vi "Matlab String(SubVI).vi"(9 "name":string, 10 "band touch win":u32(colorbox)=16734669, 11 "band touch loose":u32(colorbox)=7663) -> (3 "String":string)   [LabVIEW 2025]
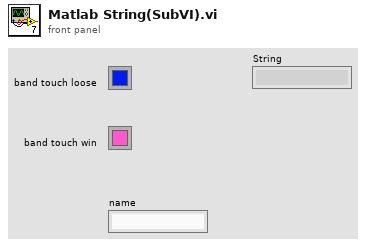
[diagram p1: front panel]
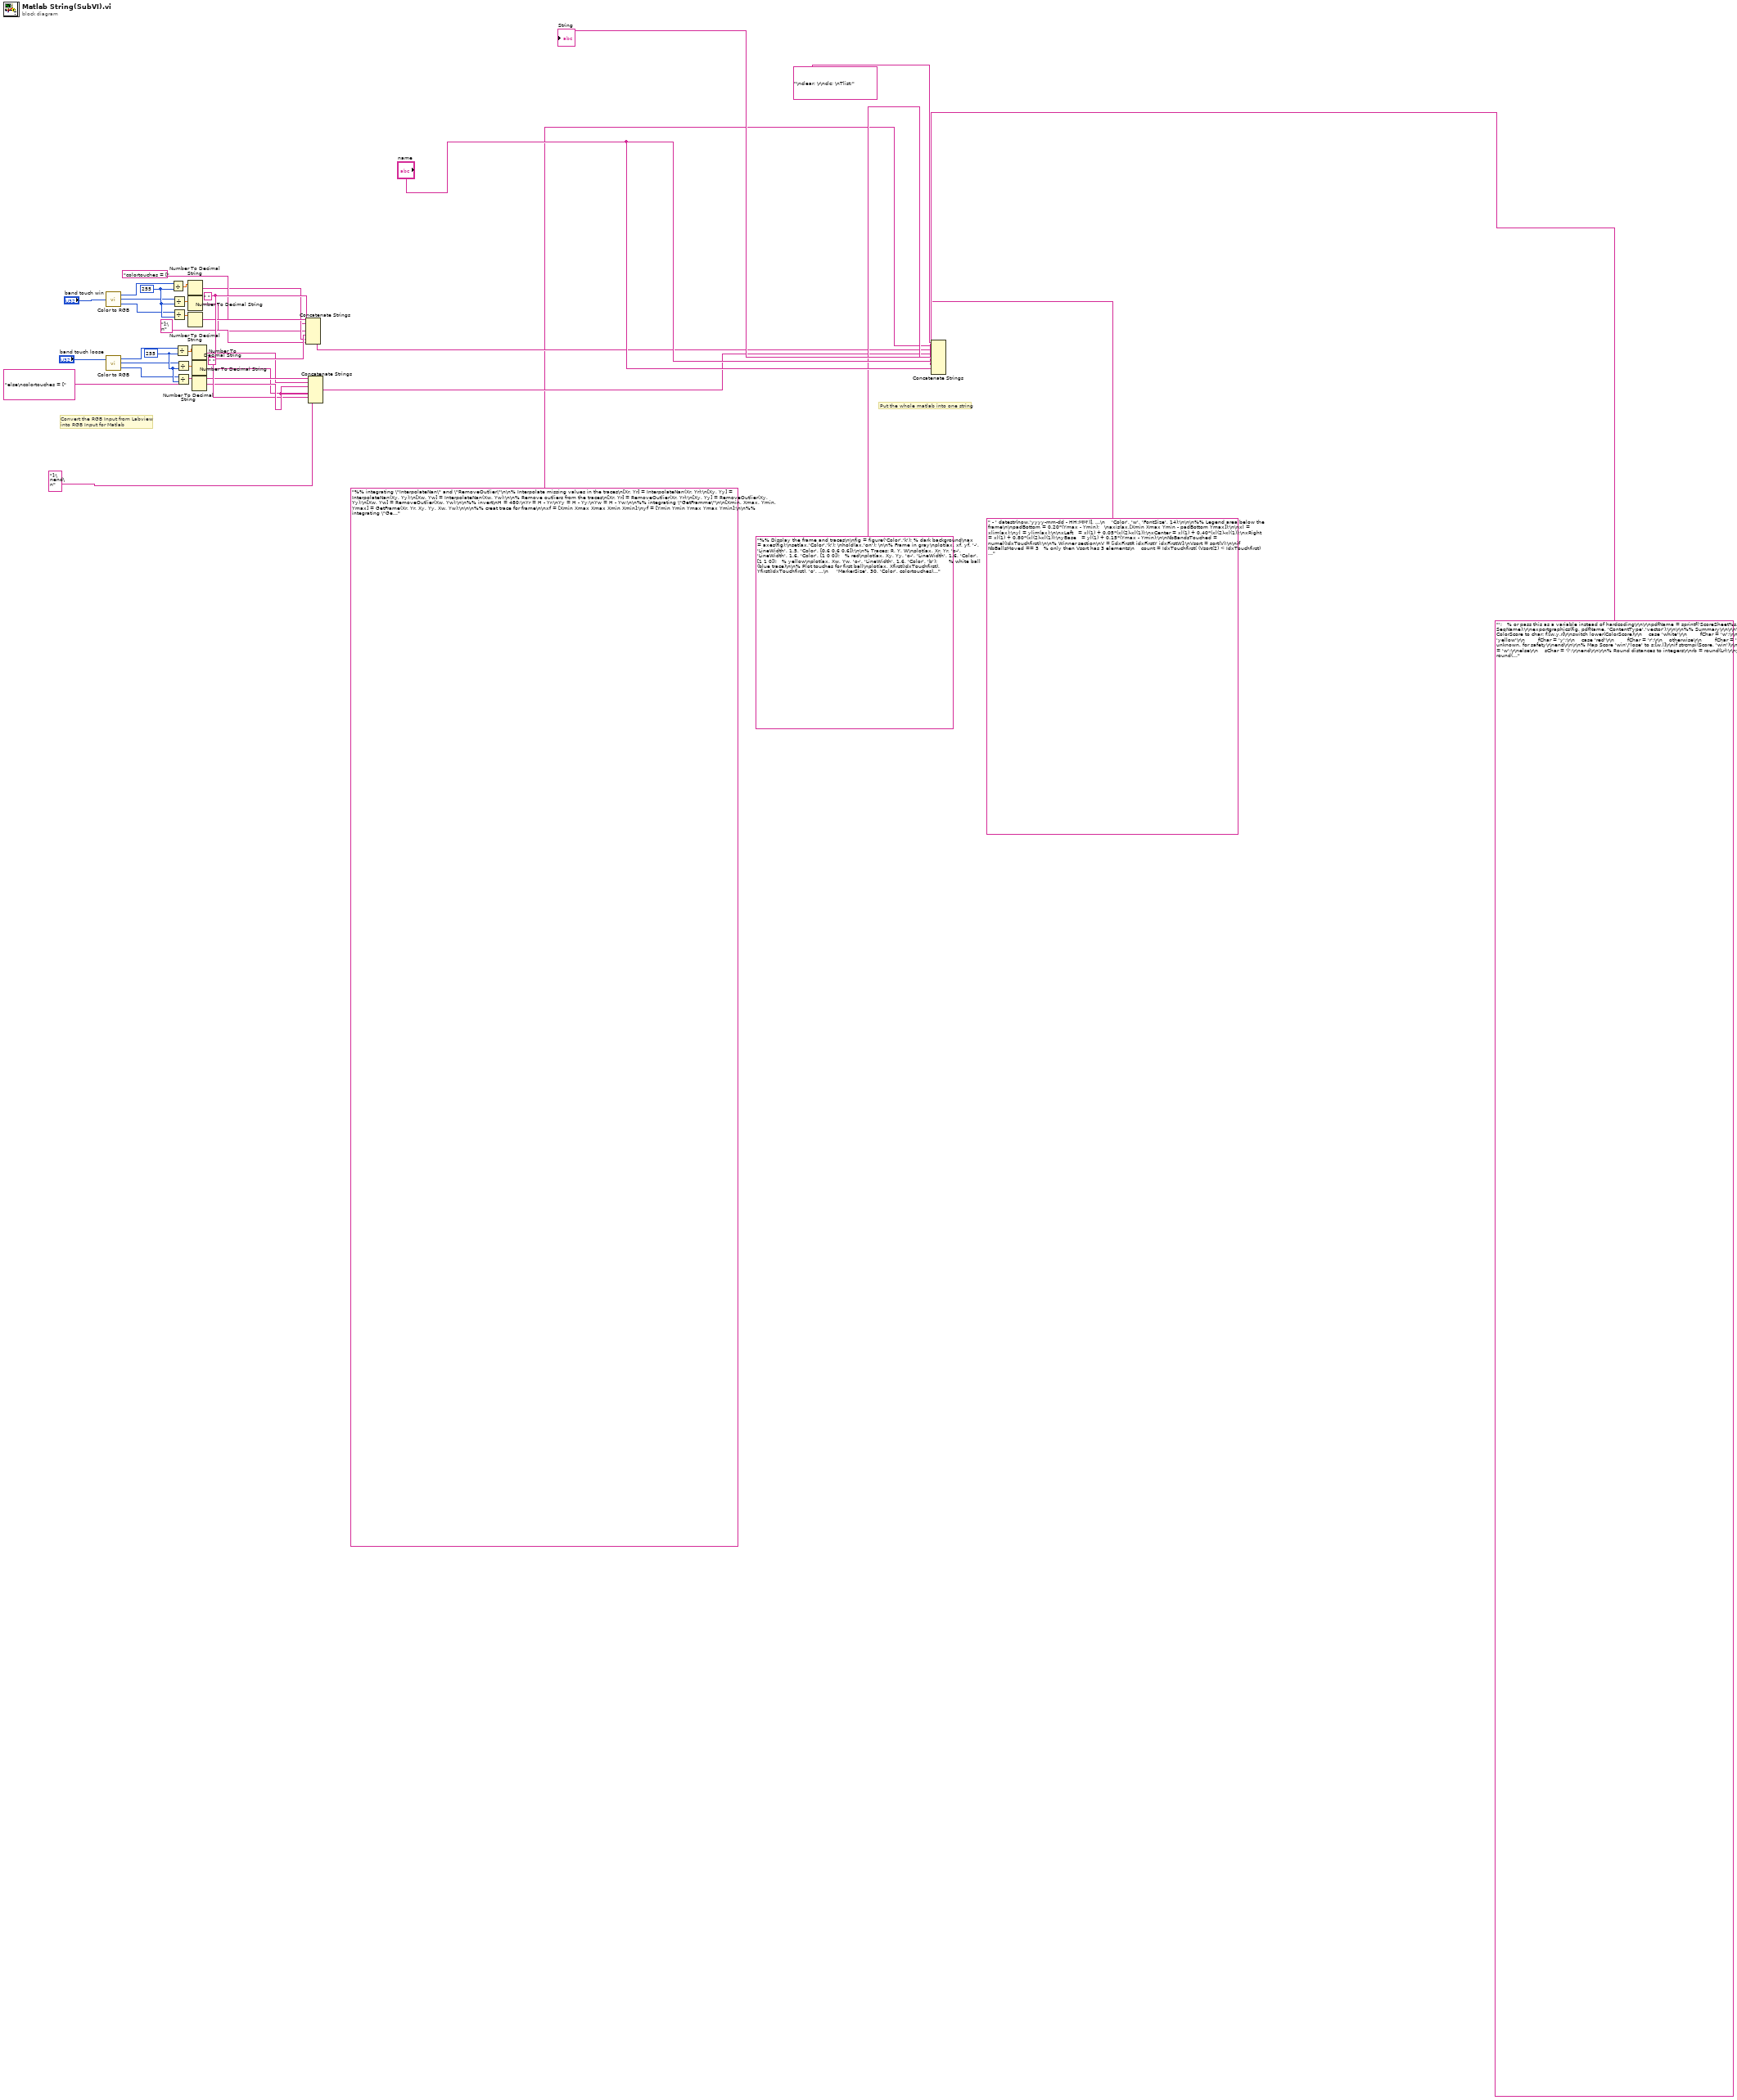
[diagram p0: block diagram]
diagram:
  w28 = " "
  w27 = 255
  w29 = " "
  w26 = 255
  # "Put the whole matlab into one string"
  # "Convert the RGB Input from Labview\ninto RGB Input for Matlab"
  n1 = call <vilib>:"Color to RGB.vi"("Color"="band touch win") -> ("R"=w22:u8, "G"=w23:u8, "B"=w24:u8)  [unwired: 1 out]
  n2 = call <vilib>:"Color to RGB.vi"("Color"="band touch loose") -> ("R"=w3:u8, "G"=w4:u8, "B"=w5:u8)  [unwired: 1 out]
  n3 = Divide(x=w22, y=w27) -> (x/y=w15:dbl)
  n4 = Divide(x=w23, y=w27) -> (x/y=w16:dbl)
  n5 = Divide(x=w24, y=w27) -> (x/y=w17:dbl)
  n6 = Divide(x=w3, y=w26) -> (x/y=w7:dbl)
  n7 = Divide(x=w4, y=w26) -> (x/y=w8:dbl)
  n8 = Divide(x=w5, y=w26) -> (x/y=w9:dbl)
  n9 = Number To Decimal String(number=w15) -> (decimal integer string=w18:string)  [unwired: 1 in]
  n10 = Number To Decimal String(number=w16) -> (decimal integer string=w19:string)  [unwired: 1 in]
  n11 = Number To Decimal String(number=w17) -> (decimal integer string=w20:string)  [unwired: 1 in]
  n12 = Number To Decimal String(number=w7) -> (decimal integer string=w10:string)  [unwired: 1 in]
  n13 = Number To Decimal String(number=w8) -> (decimal integer string=w11:string)  [unwired: 1 in]
  n14 = Number To Decimal String(number=w9) -> (decimal integer string=w12:string)  [unwired: 1 in]
  n15 = Concatenate Strings("colortouches = [" ("string"), w18, w28, w19, w28, w20, "];\n" ("string")) -> (w30:string)
  n16 = Concatenate Strings("else\ncolortouches = [" ("string"), w10, w29, w11, w29, w12, "];\nend\n" ("string")) -> (w31:string)
  n17 = Concatenate Strings("\nclear; \r\nclc; \nTlist;", "%% integrating \"InterpolateNan\" and \"RemoveOutlier\"\n\n% Interpolate missing values in the traces\n[Xr, Yr] = InterpolateNan(Xr, Yr);\n[Xy, Yy] = InterpolateNan(Xy, Yy);\n[Xw, Yw] = InterpolateNan(Xw, Yw);\n\n% Remove outliers from the traces\n[Xr, Yr] = RemoveOutlier(Xr, Yr);\n[Xy, Yy] = RemoveOutlier(Xy, Yy);\n[Xw, Yw] = RemoveOutlier(Xw, Yw);\n\n%% invert\nH = 480;\nYr = H - Yr;\nYy = H - Yy;\nYw = H - Yw;\n\n%% integrating \"GetFramme\"\n\n[Xmin, Xmax, Ymin, Ymax] = GetFrame(Xr, Yr, Xy, Yy, Xw, Yw);\n\n\n%% creat trace for frame\n\nxf = [Xmin Xmax Xmax Xmin Xmin];\nyf = [Ymin Ymin Ymax Ymax Ymin];\n\n%% integrating \"GetBallPathLength\" and \"GetFirstMoveIdx\"\nMoveDistPx = 9;\nLr = GetBallPathLength(Xr, Yr);\nLy = GetBallPathLength(Xy, Yy);\nLw = GetBallPathLength(Xw, Yw);\n\n[idxFirstR, DistMoveR] = GetFirstMoveIdx(Xr, Yr, MoveDistPx);\n[idxFirstY, DistMoveY] = GetFirstMoveIdx(Xy, Yy, MoveDistPx);\n[idxFirstW, DistMoveW] = GetFirstMoveIdx(Xw, Yw, MoveDistPx);\n\n%% integrating \"GetTouchIdx\" and \"GetBallMoveOrder\"\n\nBallBorderDist = 9;\nIdxTouchR = GetTouchIdx(Xr, Yr, Xmin, Xmax, Ymin, Ymax, BallBorderDist);\nIdxTouchY = GetTouchIdx(Xy, Yy, Xmin, Xmax, Ymin, Ymax, BallBorderDist);\nIdxTouchW = GetTouchIdx(Xw, Yw, Xmin, Xmax, Ymin, Ymax, BallBorderDist);\n\n[FirstBall, SecondBall, LastBall, NbBallsMoved] = GetBallMoveOrder(Xr, Yr, Xy, Yy, Xw, Yw, MoveDistPx);\n\nif FirstBall == 1\n    Xfirst = Xr;\n    Yfirst = Yr;\n    IdxTouchfirst = IdxTouchR;\n    ColorScore = 'red';\nelseif FirstBall == 2\n    Xfirst = Xy;\n    Yfirst = Yy;\n    IdxTouchfirst = IdxTouchY;\n    ColorScore = 'yellow';\nelse \n    Xfirst = Xw;\n    Yfirst = Yw;\n    IdxTouchfirst = IdxTouchW;\n    ColorScore = 'white';\nend\n\n%% determin Win/lose\n\nScore = GetWinnerScore(idxFirstR, idxFirstY, idxFirstW, IdxTouchfirst, NbBallsMoved);\n\nif strcmp(Score, 'win')\n    \n\n", w30, w31, "%% Display the frame and traces\n\nfig = figure('Color','k'); % dark background\nax = axes(fig);\nset(ax,'Color','k'); \nhold(ax,'on'); \n\n% Frame in gray\nplot(ax, xf, yf, '-', 'LineWidth', 1.5, 'Color', [0.6 0.6 0.6]);\n\n% Traces: R, Y, W\nplot(ax, Xr, Yr, 'o-', 'LineWidth', 1.6, 'Color', [1 0 0]);   % red\nplot(ax, Xy, Yy, 'o-', 'LineWidth', 1.6, 'Color', [1 1 0]);   % yellow\nplot(ax, Xw, Yw, 'o-', 'LineWidth', 1.6, 'Color', 'b');       % white ball (blue trace)\n\n% Plot touches for first ball\nplot(ax, Xfirst(IdxTouchfirst), Yfirst(IdxTouchfirst), 'o', ...\n     'MarkerSize', 30, 'Color', colortouches);\n\n% Plot origins\nplot(ax, Xr(1), Yr(1), 'hexagram', 'MarkerSize', 20, 'Color', [1 0 0]);\nplot(ax, Xy(1), Yy(1), 'hexagram', 'MarkerSize', 20, 'Color', [1 1 0]);\nplot(ax, Xw(1), Yw(1), 'hexagram', 'MarkerSize', 20, 'Color', 'b');\n\n% Design: frame sizing\naxis(ax,'equal');\naxis(ax,[Xmin Xmax Ymin Ymax]);\n\naxis(ax,'off');   \n\ntitle(ax, ['Scores sheet -", "name", " - ' datestr(now,'yyyy-mm-dd - HH:MM')], ...\n    'Color', 'w', 'FontSize', 14);\n\n\n%% Legend area below the frame\n\npadBottom = 0.20*(Ymax - Ymin);   \naxis(ax,[Xmin Xmax Ymin - padBottom Ymax]);\n\nxl = xlim(ax);\nyl = ylim(ax);\n\nxLeft   = xl(1) + 0.05*(xl(2)-xl(1));\nxCenter = xl(1) + 0.40*(xl(2)-xl(1));\nxRight  = xl(1) + 0.80*(xl(2)-xl(1));\nyBase   = yl(1) + 0.15*(Ymax - Ymin);\n\nNbBandsTouched = numel(IdxTouchfirst);\n\n% Winner section\nV = [idxFirstR idxFirstY idxFirstW];\nVsort = sort(V);\n\nif NbBallsMoved == 3   % only then Vsort has 3 elements\n    count = IdxTouchfirst( (Vsort(2) < IdxTouchfirst) & (IdxTouchfirst < Vsort(3)) );\n    NbBandsWin = numel(count);\nelse\n    NbBandsWin = 0;\nend\n\nif NbBallsMoved == 3 && NbBandsWin >= 3\n    Score = 'win';\nelse\n    Score = 'lose';\nend\n\n\ntext(xLeft, yBase, sprintf('Score sheet for \"%s\"', ColorScore), 'Color', 'w', 'FontSize', 12);\ntext(xLeft, yBase-30, sprintf('--- %s ---', Score), 'Color', 'w', 'FontSize', 12);\n\n% Distances\ntext(xLeft,   yBase-80, sprintf('red_d : %.0fpx',   Lr), 'Color', 'w', 'FontSize', 12);\ntext(xCenter, yBase-80, sprintf('yellow_d : %.0fpx', Ly), 'Color', 'w', 'FontSize', 12);\ntext(xRight,  yBase-80, sprintf('white_d : %.0fpx', Lw), 'Color', 'w', 'FontSize', 12);\n\n% Ball & band stats\ntext(xRight, yBase,   sprintf('%d ball(s) moved',   NbBallsMoved),   'Color', 'w', 'FontSize', 12);\ntext(xRight, yBase-30, sprintf('%d band(s) touched', NbBandsTouched), 'Color', 'w', 'FontSize', 12);\n\n%% PDF\nSeqName = '", "name", "';   % or pass this as a variable instead of hardcoding\r\n\r\npdfName = sprintf('ScoreSheet%s.pdf', SeqName);\r\nexportgraphics(fig, pdfName, 'ContentType','vector');\r\n\r\n%% Summary\r\n\r\n% Map ColorScore to char: f:[w,y,r]\r\nswitch lower(ColorScore)\r\n    case 'white'\r\n        fChar = 'w';\r\n    case 'yellow'\r\n        fChar = 'y';\r\n    case 'red'\r\n        fChar = 'r';\r\n    otherwise\r\n        fChar = 'x';   % unknown, for safety\r\nend\r\n\r\n% Map Score 'win'/'lose' to s:[w,l]\r\nif strcmpi(Score, 'win')\r\n    sChar = 'w';\r\nelse\r\n    sChar = 'l';\r\nend\r\n\r\n% Round distances to integers\r\nrb = round(Lr);\r\nyb = round(Ly);\r\nwb = round(Lw);\r\n\r\nsummaryStr = sprintf('f:%c; s:%c; n:%d; b:%d; rb:%d; yb:%d; wb:%d;', ...\r\n    fChar, sChar, NbBallsMoved, NbBandsTouched, rb, yb, wb);\r\n\r\nSummaryName = sprintf('Summary%s.txt', SeqName);\r\n\r\nfid = fopen(SummaryName, 'w');\r\nfprintf(fid, '%s\\n', summaryStr);\r\nfclose(fid);\r\n\r\n%% function InterpolateNan\r\n\r\nfunction [X, Y] = InterpolateNan(X, Y)\r\n\r\n    if isnan(X(1)),  X(1)  = 0; end\r\n    if isnan(X(end)),X(end)= 0; end\r\n\r\n    defX = ~isnan(X);\r\n    idX = 1:numel(X);\r\n    idx_defX = find(defX);\r\n    X =interp1(idx_defX,X(defX),idX,'next');\r\n\r\n    if isnan(Y(1)),  Y(1)  = 0; end\r\n    if isnan(Y(end)),Y(end)= 0; end\r\n\r\n    defY = ~isnan(Y);\r\n    idY = 1:numel(Y);\r\n    idx_defY = find(defY);\r\n    Y =interp1(idx_defY,Y(defY),idY,'next');\r\nend\r\n%% function RemoveOutlier\r\n\r\nfunction [X, Y] = RemoveOutlier(X, Y)\r\n    OX =isoutlier(X,'movmedian',10);\r\n    OY =isoutlier(Y,'movmedian',10);\r\n\r\n    O = OX & OY;\r\n    idx = find(O);\r\n    idx = idx(idx > 1);\r\n    \r\n    X(idx) = X(idx - 1);\r\n    Y(idx) = Y(idx - 1);\r\nend\r\n\r\n%% function GetFrame\r\n\r\nfunction [Xmin, Xmax, Ymin, Ymax] = GetFrame(Xr, Yr, Xy, Yy, Xw, Yw)\r\n    Xmin = min([Xr(:); Xy(:); Xw(:)], [], 'omitnan');\r\n    Xmax = max([Xr(:); Xy(:); Xw(:)], [], 'omitnan');\r\n    Ymin = min([Yr(:); Yy(:); Yw(:)], [], 'omitnan');\r\n    Ymax = max([Yr(:); Yy(:); Yw(:)], [], 'omitnan');\r\nend\r\n\r\n%% function GetBallPathLenght\r\n\r\nfunction PathLength = GetBallPathLength(X, Y)\r\n    dx = diff(X); \r\n    dy = diff(Y);\r\n    PathLength = sum( sqrt(dx.^2 + dy.^2) );\r\nend\r\n\r\n%% function GetFirstMoveIdx\r\n\r\nfunction [FirstMoveIdx, MoveDist] = GetFirstMoveIdx(X, Y, MoveDistPx)\r\n\r\n    X = X(:); \r\n    Y = Y(:);\r\n\r\n    % 1) Distances per segment \r\n    MoveDist = hypot(diff(X), diff(Y));     % length = N-1\r\n\r\n    % 2) Distance from initial position \r\n    DistFromStart = hypot(X - X(1), Y - Y(1));  % length = N\r\n\r\n    FirstMoveIdx = find(DistFromStart > MoveDistPx, 1, 'first');\r\n    if isempty(FirstMoveIdx)\r\n        FirstMoveIdx = [];  % as required: return [] if never moved\r\n    end\r\nend\r\n\r\n\r\n%% function GetTouchIdx\r\n\r\nfunction IdxTouch = GetTouchIdx(X, Y, Xmin, Xmax, Ymin, Ymax, BallBorderDist)\r\n%GETTOUCHIDX  Return time indices where the ball first touches a cushion.\r\n% A \"touch\" happens when the ball is closer than BallBorderDist to any\r\n% table border. Only the *first* index of each consecutive run is kept.\r\n\r\n    if nargin < 7 || isempty(BallBorderDist)      \nBallBorderDist = 9;            \r\n    end\r\n\r\n    % Ensure column vectors\r\n    X = X(:);  Y = Y(:);\r\n\r\n    % Logical masks: near each border\r\n    nearLeft   = (X - Xmin) < BallBorderDist;\r\n    nearRight  = (Xmax - X) < BallBorderDist;\r\n    nearBottom = (Y - Ymin) < BallBorderDist;\r\n    nearTop    = (Ymax - Y) < BallBorderDist;\r\n\r\n    % Helper: first index of every 0->1 transition (start of a \"touch\" run)\r\n    firstRunIdx = @(m) find(diff([false; m(:)]) == 1);\r\n\r\n    % Indices per border\r\n    idxL = firstRunIdx(nearLeft);\r\n    idxR = firstRunIdx(nearRight);\r\n    idxB = firstRunIdx(nearBottom);\r\n    idxT = firstRunIdx(nearTop);\r\n\r\n    % Merge borders, sort, deduplicate\r\n    IdxTouch = unique([idxL; idxR; idxB; idxT]);\r\n\r\n    % Omit index 1 if present (spec requirement)\r\n    IdxTouch(IdxTouch == 1) = [];\r\n\r\n    % If nothing touched, IdxTouch will naturally be []\r\nend\r\n\r\n%% function GetBallMoveOrder\n\nfunction [FirstBall, SecondBall, LastBall, NbBallsMoved] = ...\n    GetBallMoveOrder(Xr, Yr, Xy, Yy, Xw, Yw, MoveDistPx)\n%GETBALLMOVEORDER  Determine which ball moves first, second, and third.\n% Balls: Red=1, Yellow=2, White=3.\n%\n% Ranking rules:\n%   1) Primary key  : earliest FirstMoveIdx\n%   2) Tie-breaker  : larger first segment distance (MoveDist(1))\n%   3) Non-movers   : get index length(X)+1 (sorted to the end)\n%\n% Outputs:\n%   FirstBall, SecondBall, LastBall : labels 1/2/3\n%   NbBallsMoved : number of balls that actually moved\n\n    % --- Gather features for each ball (idx, firstSeg, len) ---\n    [idxR, segR, nR] = FirstMoveFeatures_NoNest(Xr, Yr, MoveDistPx); % Red   -> 1\n    [idxY, segY, nY] = FirstMoveFeatures_NoNest(Xy, Yy, MoveDistPx); % Yellow-> 2\n    [idxW, segW, nW] = FirstMoveFeatures_NoNest(Xw, Yw, MoveDistPx); % White -> 3\n\n    ids   = [1;      2;      3     ];\n    idxs  = [idxR;   idxY;   idxW  ];\n    segs  = [segR;   segY;   segW  ];\n    lens  = [nR;     nY;     nW    ];\n\n    % Count movers (idx <= actual length of that ball's track)\n    NbBallsMoved = sum(idxs <= lens);\n\n    % Sort by (idx ascending, firstSeg descending)\n    sortMat = [idxs, -segs];\n    [~, order] = sortrows(sortMat, [1 2]);\n\n    orderedIds = ids(order);\n\n    FirstBall  = orderedIds(1);\n    SecondBall = orderedIds(2);\n    LastBall   = orderedIds(3);\nend\n\n%% helper for GetBallMoveOrder (NOT nested)\n\nfunction [idx, firstSeg, n] = FirstMoveFeatures_NoNest(X, Y, MoveDistPx)\n%FIRSTMOVEFEATURES_NONEST Return (firstMoveIdx, firstSegmentDistance, trackLength)\n% Non-movers are assigned idx = n+1 so they sort last.\n\n    n = numel(X);\n\n    [idxFound, moveDist] = GetFirstMoveIdx(X, Y, MoveDistPx);\n\n    % Non-mover handling\n    if isempty(idxFound) || ~isfinite(idxFound) || idxFound < 1\n        idx = n + 1;   % treated as non-mover\n    else\n        idx = idxFound;\n    end\n\n    % Tie-breaker: first segment distance\n    if isempty(moveDist)\n        firstSeg = 0;\n    else\n        firstSeg = moveDist(1);\n    end\nend\n\r\n%% Winner function\r\n\r\nfunction Score = GetWinnerScore(idxFirstR, idxFirstY, idxFirstW, IdxTouchfirst, NbBallsMoved)\r\n    V = [idxFirstR idxFirstY idxFirstW];\r\n    Vsort = sort(V);\r\n    \r\n    if NbBallsMoved == 3   % only then Vsort has 3 elements\r\n        count = IdxTouchfirst(( Vsort(2) < IdxTouchfirst) & (IdxTouchfirst < Vsort(3)) );\r\n        NbBandsWin = numel(count);\r\n    else\r\n        NbBandsWin = 0;\r\n    end\r\n    \r\n    if NbBallsMoved == 3 && NbBandsWin >= 3\r\n        Score = 'win';\r\n    else\r\n        Score = 'lose';\r\n    end\r\nend\n") -> (→"String":string)
